vi "test place in stack.vi"() -> ()   [LabVIEW 2018]
panel:
  in  "c1":dbl
  in  "c2":dbl
  in  "stop":bool
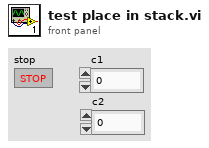
[diagram p1: front panel]
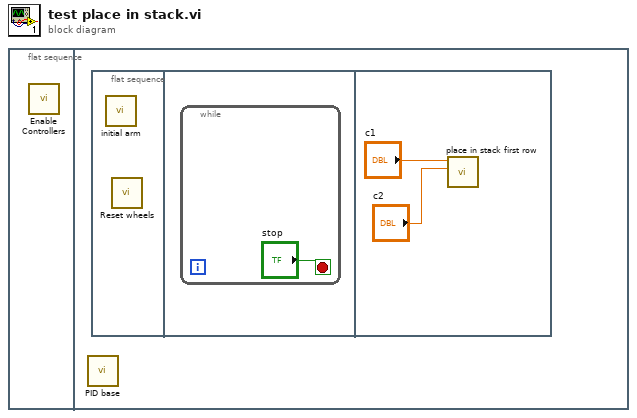
[diagram p0: block diagram]
diagram:
  n1 = flat-sequence {
    frame #0 {
      n2 = call "Enable Controllers.vi"() -> ()  [unwired: 12 in]
    }
    frame #1 {
      n3 = call "PID base.vi"() -> ()  [unwired: 12 in]
      n4 = flat-sequence {
        frame #0 {
          n5 = call "initial arm.vi"() -> ()  [unwired: 12 in]
          n6 = call "Reset wheels.vi"() -> ()  [unwired: 12 in]
        }
        frame #1 {
          n7 = while {
            stop <- "stop" stop-if-true
          }
        }
        frame #2 {
          n8 = call "place in stack first row.vi"("c2"="c2", "c1"="c1") -> ()  [unwired: 10 in]
        }
      }
    }
  }
